vi "Disonnect Trigger Terminals-Array.vi"(8 "error in (no error)":errorcluster, 10 "Routing Information":T1[](array[typedef]), 11 "instrument handle":refnum<k15>) -> (0 "error out":errorcluster, 3 "instrument handle out":refnum<k15>)   [LabVIEW 2026]
doc: "This VI allows an array input of Trigger Routing Controls. NI-SYNC will make the disconnects of each array input. The benefit of this vi is there is no need for multiple string inputs."
uses:
  Trigger Routing.ctl
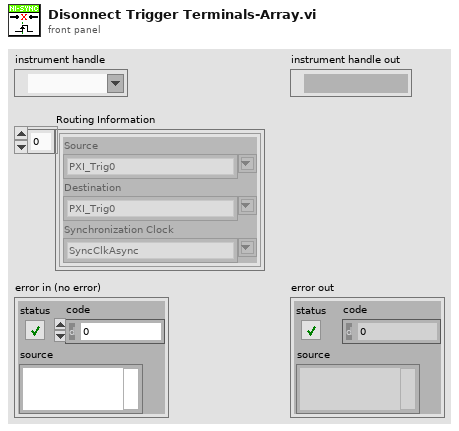
[diagram p1: front panel]
types:
  T1 = typedef "Trigger Routing.ctl" = cluster{"Source":string, "Destination":string, "Synchronization Clock":string}
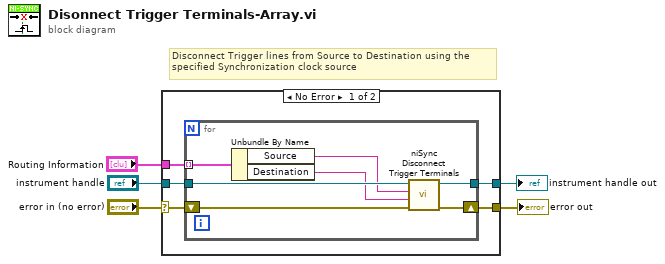
[diagram p0: block diagram]
diagram:
  # "Disconnect Trigger lines from Source to Destination using the\nspecified Synchronization clock source"
  n1 = case shown="No Error" "error in (no error)" {
    selector: "error in (no error)" -> [w7 w19]
    tunnel: "Routing Information" -> [w10 _]
    tunnel: "instrument handle" -> [w9 w18]
    tunnel: [w8 w18] -> w5
    tunnel: [w6 w19] -> w3
    frame No Error {
      n2 = for {
        tunnel: w9 -> [w17]
        shift-right: [w15] -> w6
        shift-left: w7 -> [w16]
        tunnel: w10 -> [w14] mode=indexing
        tunnel: [w11] -> w8
        n3 = Unbundle By Name(w14) -> ("Source"=w13:string, "Destination"=w12:string)
        n4 = call <instrlib>:"niSync Disconnect Trigger Terminals.vi"("error in (no error)"=w16, "destination terminal"=w12, "source terminal"=w13, "instrument handle"=w17) -> ("error out"=w15:errorcluster, "instrument handle out"=w11:refnum<k15>)  [unwired: 6 in]
      }
    }
    frame Error {
    }
  }
  "instrument handle out" <- w5
  "error out" <- w3
